vi "send_data.vi"(8 "error in (no error)":errorcluster, 10 "send data (string)":string) -> (0 "error out":errorcluster, 2 "timeout?":bool)   [LabVIEW 2016, in "BT-Android_interface.lvlib"]
uses:
  BT-Android_interface.lvlib
  mode.ctl
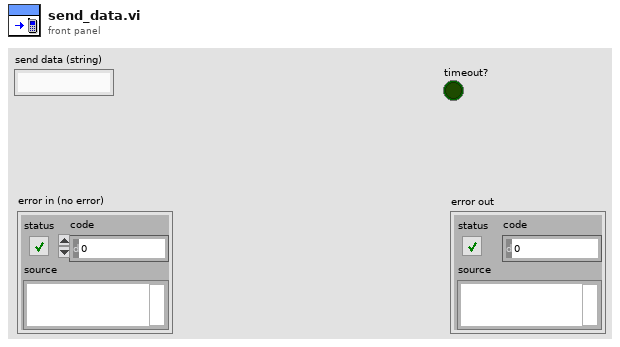
[diagram p1: front panel]
types:
  T1 = typedef "BT-Android_interface.lvlib/mode.ctl" = enum16{"init", "broadcast_data", "receive_data", "close"}
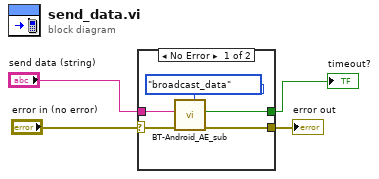
[diagram p0: block diagram]
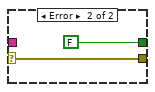
[diagram p2: hidden frame]
diagram:
  n1 = case shown="No Error" "error in (no error)" {
    selector: "error in (no error)" -> [w9 w11]
    tunnel: [w8 w11] -> w3
    tunnel: "send data (string)" -> [w7 _]
    tunnel: [w6 FALSE ("timeout?")] -> w1
    frame No Error {
      n2 = call "BT-Android_AE_sub.vi"("mode"=mode."broadcast_data", "error in (no error)"=w9, "send data"=w7) -> ("error IO"=w8:errorcluster, "timeout?"=w6:bool)  [unwired: 7 in]
    }
    frame Error {
    }
  }
  "error out" <- w3
  "timeout?" <- w1
